vi "_CH375_Get.vi"(8 "Error In":errorcluster caption="错误输入") -> (0 "Error Out":errorcluster caption="错误输出", 3 "实时角度(参考值)":dbl)   [LabVIEW 2020, in "CH375.lvlib"]
uses:
  CH375.lvlib
  CH375DLL64.dll
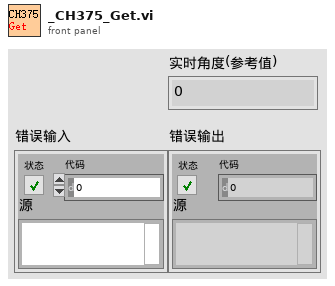
[diagram p1: front panel]
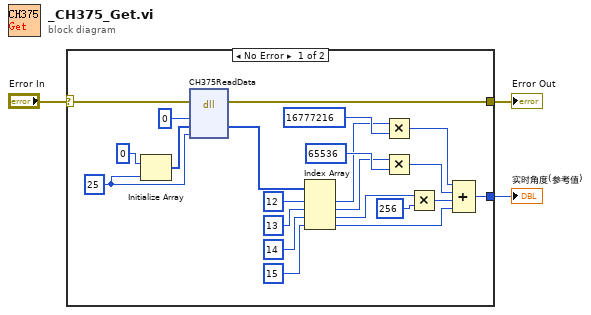
[diagram p0: block diagram]
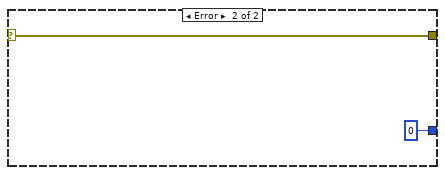
[diagram p2: hidden frame]
diagram:
  n1 = case shown="No Error" "Error In" {
    selector: "Error In" -> [w9 w27]
    tunnel: [w10 w27] -> w2
    tunnel: [w8 0] -> w1
    frame No Error {
      w12 = 25 ("维数大小")
      n2 = Initialize Array(u8 0 ("元素"), w12) -> (w21:u8[])
      n3 = dll-call lib="D:/Project NJU/lib/CH375/CH375DLL64.dll" fn="CH375ReadData" label="中断读数据"(error in=w9, "index"=u32 0, "buff"=w21, "length"=w12) -> (error out=w10:errorcluster, "buff"=w22:u8[])  [unwired: 3 in, 3 out]
      n4 = Index Array(array=w22, index #1=12 ("索引"), index #2=13 ("索引"), index #3=14 ("索引"), index #4=15 ("索引")) -> (element #1=w7:u8, element #2=w6:u8, element #3=w5:u8, element #4=w4:u8)
      n5 = Multiply(x=w7, y=16777216) -> (x*y=w23:i32)
      n6 = Multiply(x=w6, y=65536) -> (x*y=w24:i32)
      n7 = Multiply(x=w5, y=256) -> (x*y=w25:i32)
      n8 = Compound Arithmetic op=ADD(w23, w24, w25, w4) -> (w8:i32)
    }
    frame Error {
    }
  }
  "Error Out" <- w2
  "实时角度(参考值)" <- w1
